vi "create.vi"(8 "error in (no error)":errorcluster, 11 "Type":T1(ring)=enum."SCOPE_NI") -> (0 "error out":errorcluster, 3 "Scope.lvclass":refnum<class "Scope.lvclass">)   [LabVIEW 2023, in "sweScope.lvlib" / "Scope.lvclass"]
doc: "Create a new scope object."
uses:
  Scope.lvclass
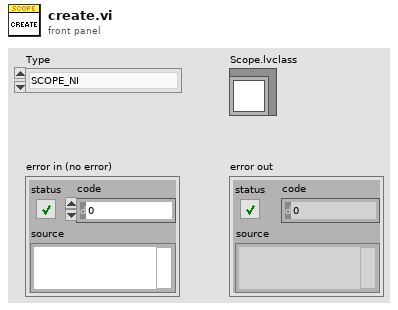
[diagram p1: front panel]
types:
  T1 = enum16{"Simulated", "SCOPE_NI", "SCOPE_Keysight"}
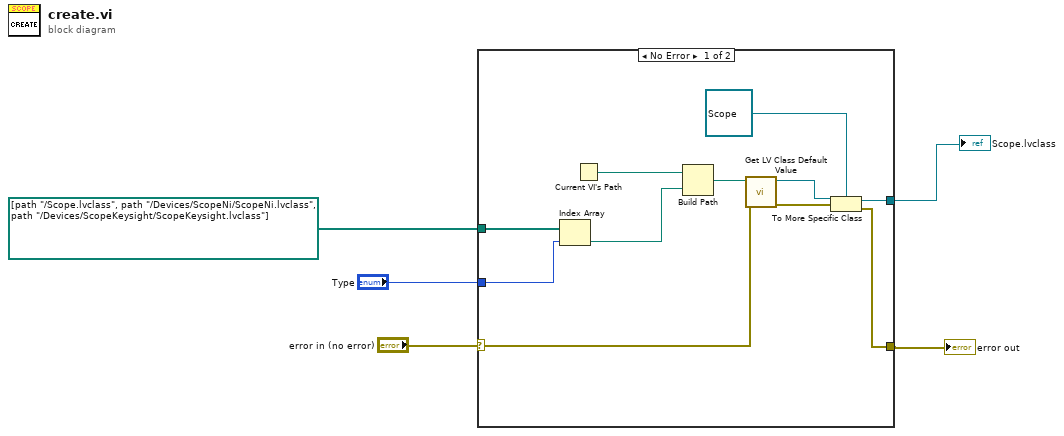
[diagram p0: block diagram]
diagram:
  n1 = case shown="No Error" "error in (no error)" {
    selector: "error in (no error)" -> [w15 w17]
    tunnel: [w13 _] -> w5
    tunnel: path[] [path "../Scope.lvclass", path "../Devices/ScopeNi/ScopeNi.lvclass", path "../Devices/ScopeKeysight/ScopeKeysight.lvclass"] ("Relative Paths") -> [w12 _]
    tunnel: "Type" -> [w10 _]
    tunnel: [w7 w17] -> w4
    frame No Error {
      n2 = Index Array(array=w12, index=w10) -> (element=w11:path)
      n3 = Current VI's Path() -> (path=w16:path)
      n4 = Build Path(base path=w16, name or relative path=w11) -> (appended path=w14:path)
      n5 = call <vilib>:"Get LV Class Default Value.vi"("error in (no error)"=w15, "class path"=w14) -> ("error out"=w9:errorcluster, "object"=w8:refnum<class>)  [unwired: 8 in]
      n6 = To More Specific Class(target class=refnum<class "Scope.lvclass"> refnum ("Fgen.lvclass"), reference=w8, error in=w9) -> (specific class reference=w13:refnum<class "Scope.lvclass">, error out=w7:errorcluster)
    }
    frame Error {
    }
  }
  "Scope.lvclass" <- w5
  "error out" <- w4
